vi "Update Fan.vi"(8 "error in (no error)":errorcluster caption="entrée d'erreur (pas d'erreur)", 9 "Fan B":cluster{"State":bool, "Fault":bool}, 10 "Fan A":cluster{"State":bool, "Fault":bool}, 11 "Cooler UI with Events en entrée":refnum<class "Cooler UI with Events.lvclass">) -> (0 "error out":errorcluster caption="sortie d'erreur", 3 "Cooler UI with Events en sortie":refnum<class "Cooler UI with Events.lvclass">)   [LabVIEW 2015, in "Cooler UI.lvlib" / "Cooler UI with Events.lvclass"]
uses:
  Cooler UI with Events.lvclass
  Cooler UI with Events.lvclass/Cooler UI with Events.ctl
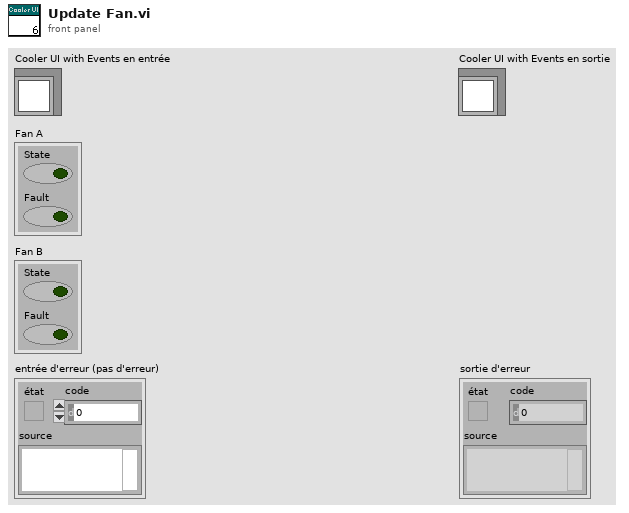
[diagram p1: front panel]
types:
  T1 = cluster{"Fan A":cluster{"State":bool, "Fault":bool}, "Fan B":cluster{"State":bool, "Fault":bool}}
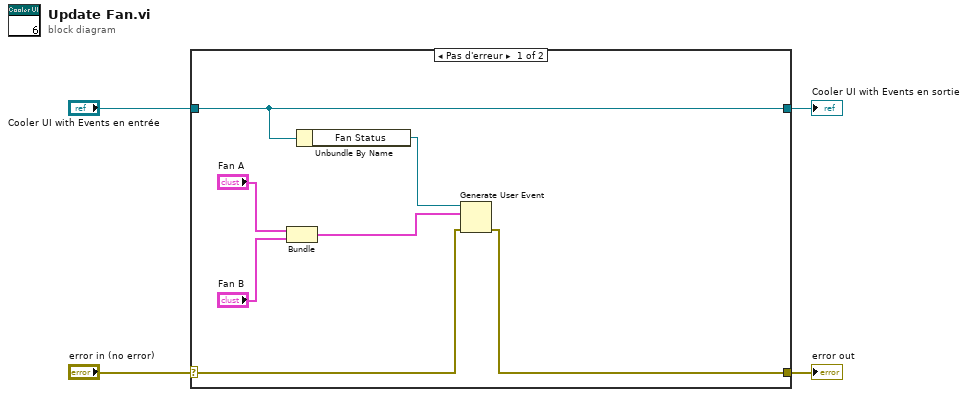
[diagram p0: block diagram]
diagram:
  n1 = case shown="Pas d'erreur" "error in (no error)" {
    selector: "error in (no error)" -> [w6 w13]
    tunnel: [w5 w13] -> w3
    tunnel: [w9 w12] -> w1
    tunnel: "Cooler UI with Events en entrée" -> [w9 w12]
    frame No Error {
      n2 = Bundle("Fan A"="Fan A", "Fan B"="Fan B") -> (w7:T1)  [unwired: 1 in]
      n3 = Unbundle By Name(w9) -> ("Fan Status"=w8:refnum<user-event>)
      n4 = Generate User Event(user event=w8, event data cluster=w7, error in=w6) -> (error out=w5:errorcluster)  [unwired: 1 in, 1 out]
    }
    frame Error {
    }
  }
  "error out" <- w3
  "Cooler UI with Events en sortie" <- w1
